vi "SortTemplates.vi"(11 "Unsorted Templates":refnum<class "MetaDataObj.lvclass">[](array[class])) -> (3 "Sorted Templates":refnum<class "MetaDataObj.lvclass">[](array[class]))   [LabVIEW 2016]
uses:
  <resource>/dialog/NewProjectWizard/MetaDataObj/MetaDataObj.lvclass
  <resource>/dialog/NewProjectWizard/MetaDataObj/Accessors/Read Sort Priority.vi
  <resource>/dialog/NewProjectWizard/MetaDataObj/Accessors/Read Title.vi
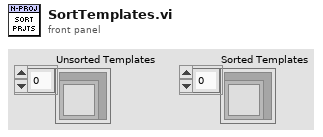
[diagram p1: front panel]
types:
  T1 = cluster{"Sort Priority":dbl, string, "Template":refnum<class "MetaDataObj.lvclass">}
  T2 = cluster{"Sort Priority":dbl, string, "Template":refnum<class "MetaDataObj.lvclass">}[]
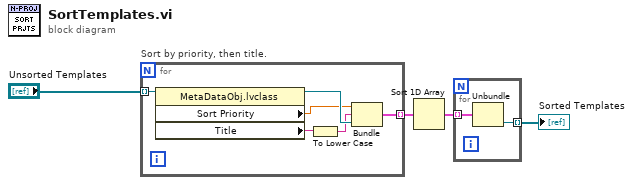
[diagram p0: block diagram]
diagram:
  n1 = for "Sort by priority, then title." {
    tunnel: "Unsorted Templates" -> [w10] mode=indexing
    tunnel: [w9] -> w3 mode=indexing
    n2 = property class="MetaDataObj.lvclass"(reference=w10) -> (reference out=w7:refnum<class "MetaDataObj.lvclass">, "Sort Priority"=w5:dbl, "Title"=w8:string)  [unwired: 1 in, 1 out]
    n3 = To Lower Case(string=w8) -> (all lower case string=w6:string)
    n4 = Bundle("Sort Priority"=w5, w6, "Template"=w7) -> (w9:T1)  [unwired: 1 in]
  }
  n5 = Sort 1D Array(array=w3) -> (sorted array=w2:T2)
  n6 = for {
    tunnel: w2 -> [w12] mode=indexing
    tunnel: [w11] -> w1 mode=indexing
    n7 = Unbundle(w12) -> ("Template"=w11:refnum<class "MetaDataObj.lvclass">)  [unwired: 2 out]
  }
  "Sorted Templates" <- w1
